vi "viewer3.vi"() -> (8 "cloudRGB_source":u32[](array[numeric]), 9 "cloudZ_source":sgl[](array[numeric]), 10 "cloudY_source":sgl[](array[numeric]), 11 "cloudX_source":sgl[](array[numeric]))   [LabVIEW 2012]
uses:
  G_SEN.vi
  G_NAV.vi
  dlls/PCL_OpenCV_LabviewToolkit_visualize_redraw.dll
panel:
  out "processing time [ms]":u32=43
  out "transformation_matrix":sgl[][](array[numeric])=[[1.0000002, 2.1462839e-07, -1.6423296e-07, 0.7000001], [-1.3767561e-07, 1.0, -6.5921284e-08, -7.4505806e-08], [1.6773438e-07, 2.9214991e-08, 1.0, 9.313226e-08], [0.0, 0.0, 0.0, 1.0]]
  out "TMP":dbl[][](array[numeric])=[[-1.989725401977954, 16.427453516317758, 0.5413148846973371]]
  out "x-y":u32
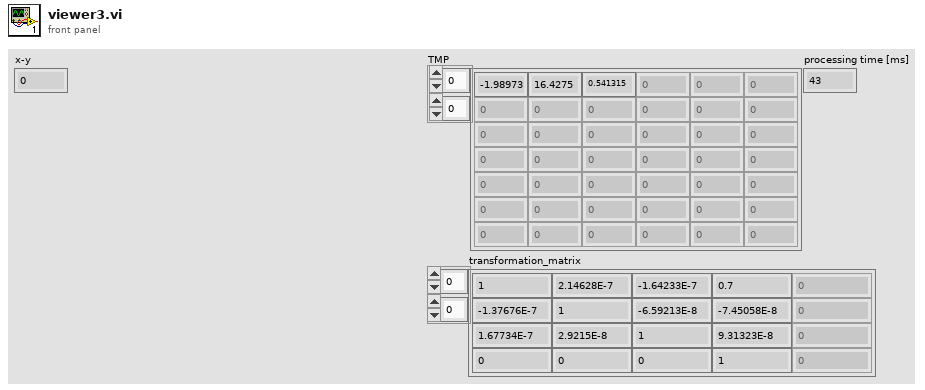
[diagram p1: front panel]
types:
  T1 = cluster{"GPSTime":dbl, "attitude[2]":dbl, "lcc[0]":dbl, "lcc[1]":dbl, "heading_GPS":dbl}
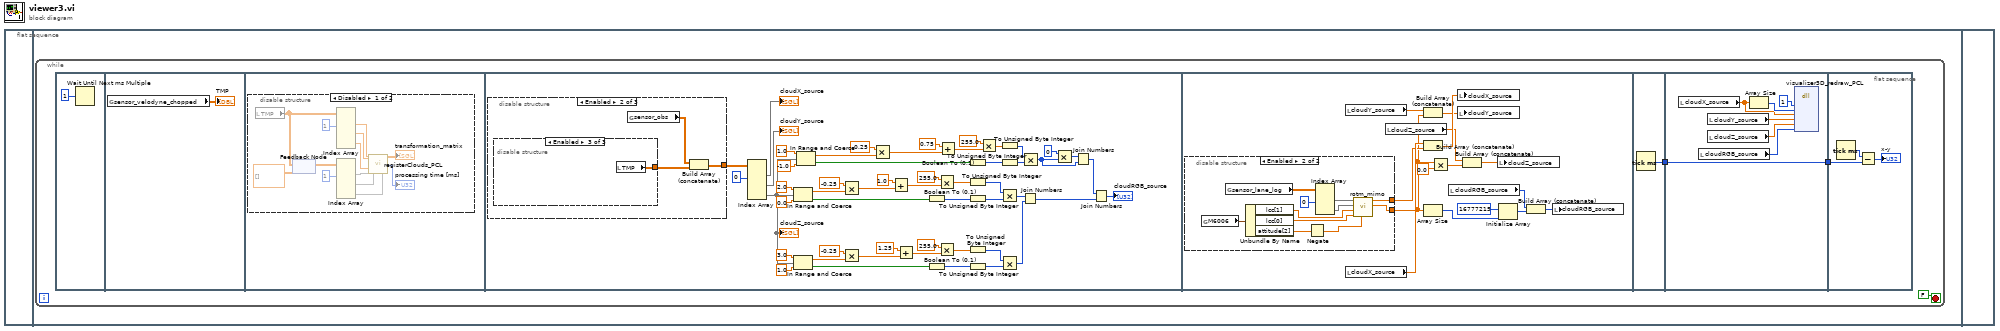
[diagram p0: block diagram]
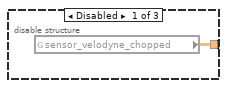
[diagram p3: hidden frame]
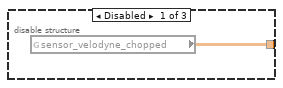
[diagram p4: hidden frame]
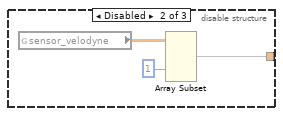
[diagram p5: hidden frame]
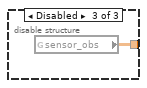
[diagram p6: hidden frame]
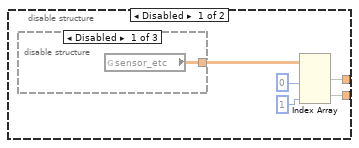
[diagram p7: hidden frame]
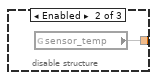
[diagram p8: hidden frame]
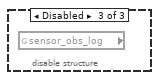
[diagram p9: hidden frame]
diagram:
  n1 = flat-sequence {
    frame #0 {
    }
    frame #1 {
      n2 = while {
        stop <- FALSE stop-if-true
        n3 = flat-sequence {
          tunnel: [w114] -> w1
          tunnel: w1 -> [w119]
          tunnel: [w119] -> w2
          tunnel: w2 -> [w123]
          frame #0 {
            n4 = Wait Until Next ms Multiple(millisecond multiple=u32 1) -> ()  [unwired: 1 out]
          }
          frame #1 {
            n5 = global read "G_SEN.vi" "sensor_velodyne_chopped"() -> (→"TMP":dbl[][])
          }
          frame #2 {
            n6 = disable-structure shown="Disabled" {
              frame Disabled {
                n7 = local read "TMP"() -> (w11:dbl[][])
                n8 = feedback #1(dbl[][] [] ("TMP")) -> (w17:dbl[][])
                n9 = feedback-in #1(w11) -> ()
                n10 = Index Array(array=w11, index (col) #1=1 ("disabled index (col)")) -> (element #1=w10:dbl[], element #2=w9:dbl[], element #3=w8:dbl[])  [unwired: 5 in]
                n11 = Index Array(array=w17, index (col) #1=1 ("disabled index (col)")) -> (element #1=w15:dbl[], element #2=w14:dbl[], element #3=w13:dbl[])  [unwired: 5 in]
                n12 = call "registerClouds_PCL.vi"("cloudX_target"=w10, "cloudY_target"=w9, "cloudZ_target"=w8, "cloudX_source"=w15, "cloudY_source"=w14, "cloudZ_source"=w13) -> ("transformation_matrix"=→"transformation_matrix":sgl[][], "processing time [ms]"=→"processing time [ms]":u32)  [unwired: 16 in, 4 out]
              }
              frame Enabled {
              }
            }
          }
          frame #3 {
            n13 = disable-structure shown="Enabled" {
              disable-tunnel: [w71 w72 w80] -> w70
              frame Disabled {
                n14 = global read "G_SEN.vi" "sensor_velodyne_chopped"() -> (w71:dbl[][])
              }
              frame Enabled {
                n15 = disable-structure shown="Enabled" {
                  disable-tunnel: [w75 w77 w79] -> w73
                  frame Disabled {
                    n16 = global read "G_SEN.vi" "sensor_velodyne_chopped"() -> (w75:dbl[][])
                  }
                  frame Disabled {
                    n17 = global read "G_SEN.vi" "sensor_velodyne"() -> (w78:dbl[][])
                    n18 = Array Subset(array=w78, index (col)=1 ("index")) -> (w77:dbl[][])  [unwired: 3 in]
                  }
                  frame Enabled {
                    n19 = local read "TMP"() -> (w79:dbl[][])
                  }
                }
                n20 = global read "G_SEN.vi" "sensor_obs"() -> (w74:dbl[][])
                n21 = Build Array (concatenate)(w74, w73) -> (w72:dbl[][])
              }
              frame Disabled {
                n22 = global read "G_SEN.vi" "sensor_obs"() -> (w80:dbl[][])
              }
            }
            n23 = Index Array(array=w70, index (col) #1=0 ("disabled index (col)")) -> (element #1=→"cloudX_source":dbl[], element #2=→"cloudY_source":dbl[], element #3=w20:dbl[])  [unwired: 5 in]
            "cloudZ_source" <- w20
            n24 = In Range and Coerce(upper limit=2.0, x=w20, lower limit=0.0) -> (coerced(x)=w63:dbl[], In Range?=w34:bool[])
            n25 = In Range and Coerce(upper limit=3.0, x=w20, lower limit=1.0) -> (coerced(x)=w66:dbl[], In Range?=w26:bool[])
            n26 = In Range and Coerce(upper limit=1.0, x=w20, lower limit=-1.0) -> (coerced(x)=w51:dbl[], In Range?=w50:bool[])
            n27 = Multiply(x=-0.25, y=w63) -> (x*y=w53:dbl[])
            n28 = Multiply(x=-0.25, y=w66) -> (x*y=w55:dbl[])
            n29 = Multiply(x=-0.25, y=w51) -> (x*y=w57:dbl[])
            n30 = Add(x=1.0, y=w53) -> (x+y=w35:dbl[])
            n31 = Add(x=1.25, y=w55) -> (x+y=w27:dbl[])
            n32 = Boolean To (0,1)(Boolean=w34) -> (0, 1=w39:i16[])
            n33 = Boolean To (0,1)(Boolean=w26) -> (0, 1=w30:i16[])
            n34 = Multiply(x=255.0, y=w35) -> (x*y=w37:dbl[])
            n35 = Multiply(x=255.0, y=w27) -> (x*y=w32:dbl[])
            n36 = Add(x=0.75, y=w57) -> (x+y=w49:dbl[])
            n37 = Boolean To (0,1)(Boolean=w50) -> (0, 1=w45:i16[])
            n38 = To Unsigned Byte Integer(number=w37) -> (unsigned 8bit integer=w38:u8[])
            n39 = To Unsigned Byte Integer(number=w39) -> (unsigned 8bit integer=w40:u8[])
            n40 = To Unsigned Byte Integer(number=w32) -> (unsigned 8bit integer=w31:u8[])
            n41 = To Unsigned Byte Integer(number=w30) -> (unsigned 8bit integer=w29:u8[])
            n42 = Multiply(x=255.0, y=w49) -> (x*y=w47:dbl[])
            n43 = To Unsigned Byte Integer(number=w47) -> (unsigned 8bit integer=w46:u8[])
            n44 = To Unsigned Byte Integer(number=w45) -> (unsigned 8bit integer=w44:u8[])
            n45 = Multiply(x=w38, y=w40) -> (x*y=w25:u8[])
            n46 = Multiply(x=w31, y=w29) -> (x*y=w28:u8[])
            n47 = Multiply(x=w46, y=w44) -> (x*y=w43:u8[])
            n48 = Join Numbers(hi=w25, lo=w28) -> ((hi.lo)=w23:u16[])
            n49 = Multiply(x=u8 0, y=w43) -> (x*y=w41:u8[])
            n50 = Join Numbers(hi=w41, lo=w43) -> ((hi.lo)=w24:u16[])
            n51 = Join Numbers(hi=w24, lo=w23) -> ((hi.lo)=→"cloudRGB_source":u32[])
          }
          frame #4 {
            n52 = disable-structure shown="Enabled" {
              disable-tunnel: [w100 w103] -> w86
              disable-tunnel: [w99 w104] -> w94
              frame Disabled {
                n53 = disable-structure shown="Disabled" {
                  disable-tunnel: [w101 w102 _] -> w98
                  frame Disabled {
                    n54 = global read "G_SEN.vi" "sensor_etc"() -> (w101:dbl[][])
                  }
                  frame Enabled {
                    n55 = global read "G_SEN.vi" "sensor_temp"() -> (w102)
                  }
                  frame Disabled {
                    n56 = global read "G_SEN.vi" "sensor_obs_log"() -> ()  [unwired: 1 out]
                  }
                }
                n57 = Index Array(array=w98, index (col) #1=0 ("disabled index (col)"), index (col) #2=1 ("index (col)")) -> (element #1=w99:dbl[], element #2=w100:dbl[])  [unwired: 2 in]
              }
              frame Enabled {
                n58 = global read "G_NAV.vi" "M6006"() -> (w107:T1)
                n59 = global read "G_SEN.vi" "sensor_lane_log"() -> (w112:dbl[][])
                n60 = Unbundle By Name(w107) -> ("lcc[1]"=w111:dbl, "lcc[0]"=w110:dbl, "attitude[2]"=w109:dbl)
                n61 = Negate(x=w109) -> (-x=w108:dbl)
                n62 = Index Array(array=w112, index (col) #1=0 ("disabled index (col)")) -> (element #1=w106:dbl[], element #2=w105:dbl[])  [unwired: 3 in]
                n63 = call "rotm_mimo.vi"("angle[rad]"=w108, "y0"=w110, "x0"=w111, "y"=w105, "x"=w106) -> ("Y"=w103:dbl[], "X"=w104:dbl[])  [unwired: 3 in, 2 out]
              }
            }
            n64 = local read "cloudY_source"() -> (w91:sgl[])
            n65 = local read "cloudX_source"() -> (w95:sgl[])
            n66 = local read "cloudZ_source"() -> (w90:sgl[])
            n67 = Build Array (concatenate)(w91, w86) -> (w92:dbl[])
            n68 = Build Array (concatenate)(w95, w94) -> (w93:dbl[])
            n69 = Array Size(array=w86) -> (size(s)=w85:i32)
            n70 = Multiply(x=w86, y=0.0) -> (x*y=w87:dbl[])
            n71 = local read "cloudRGB_source"() -> (w83:u32[])
            n72 = local write "cloudX_source"(w93) -> ()
            n73 = local write "cloudY_source"(w92) -> ()
            n74 = Build Array (concatenate)(w90, w87) -> (w89:dbl[])
            n75 = local write "cloudZ_source"(w89) -> ()
            n76 = Initialize Array(u32 16777215 ("(hi.lo)"), w85) -> (w82:u32[])
            n77 = Build Array (concatenate)(w83, w82) -> (w81:u32[])
            n78 = local write "cloudRGB_source"(w81) -> ()
          }
          frame #5 {
            n79 = Tick Count (ms)() -> (millisecond timer value=w114:u32)
          }
          frame #6 {
            n80 = local read "cloudX_source"() -> (w118:sgl[])
            n81 = local read "cloudRGB_source"() -> (w115:u32[])
            n82 = local read "cloudY_source"() -> (w117:sgl[])
            n83 = local read "cloudZ_source"() -> (w116:sgl[])
            n84 = Array Size(array=w118) -> (size(s)=w121:i32)
            n85 = dll-call lib="C:/eurecar/3d/dlls/PCL_OpenCV_LabviewToolkit_visualize_redraw.dll" fn="visualizer3D_redraw_PCL"("cloudCols_source"=1, "cloudRows_source"=w121, "cloudX_source"=w118, "cloudY_source"=w117, "cloudZ_source"=w116, "cloudRGB_source"=w115) -> ()  [unwired: 10 in, 2 out]
          }
          frame #7 {
            n86 = Tick Count (ms)() -> (millisecond timer value=w124:u32)
            n87 = Subtract(x=w124, y=w123) -> (x-y=→"x-y":u32)
          }
        }
      }
    }
    frame #2 {
    }
  }
